vi "Parse Spreadsheet Array.vi"(11 "all rows":dbl[][](array[numeric])) -> (0 "Projectile Velocity (m/s)":dbl, 1 "Strain Amplifier (Volts)":dbl[](array[numeric]), 2 "Time (Seconds)":dbl[](array[numeric]), 3 "Waveform":waveform(dbl))   [LabVIEW 2020]
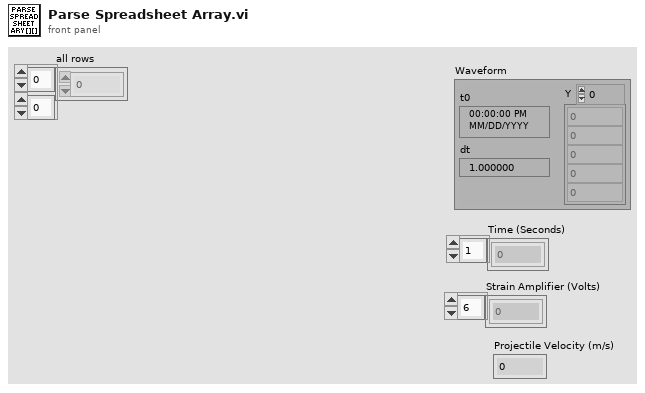
[diagram p1: front panel]
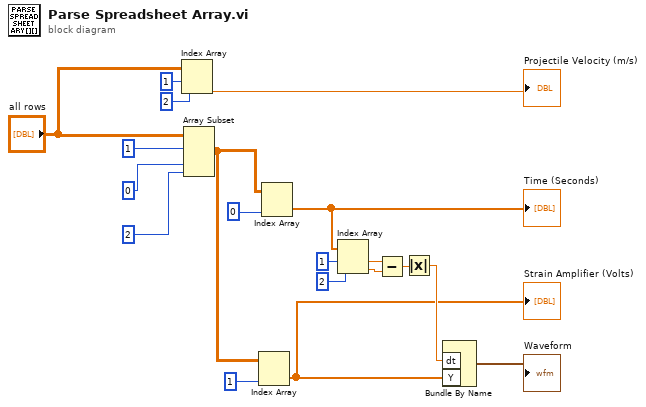
[diagram p0: block diagram]
diagram:
  n1 = Index Array(array="all rows", index (row)=1, index (col)=2 ("disabled index (col)")) -> (element=→"Projectile Velocity (m/s)":dbl)
  n2 = Array Subset(array="all rows", index (row)=1 ("index"), index (col)=0 ("index"), length (col)=2 ("length")) -> (w4:dbl[][])  [unwired: 1 in]
  n3 = Index Array(array=w4, index (col)=1 ("index (row)")) -> (element=w11:dbl[])  [unwired: 1 in]
  "Strain Amplifier (Volts)" <- w11
  n4 = Index Array(array=w4, index (col)=0 ("index (row)")) -> (element=w12:dbl[])  [unwired: 1 in]
  "Time (Seconds)" <- w12
  n5 = Index Array(array=w12, index #1=1 ("index"), index #2=2 ("index")) -> (element #1=w15:dbl, element #2=w16:dbl)
  n6 = Subtract(x=w15, y=w16) -> (x-y=w18:dbl)
  n7 = Absolute Value(x=w18) -> (abs(x)=w19:dbl)
  n8 = Bundle By Name("dt"=w19, "Y"=w11) -> (→"Waveform":waveform(dbl))  [unwired: 1 in]
